vi "GetBit.vi"(8 "error in (no error)":errorcluster, 10 "Index":i32, 11 "Prime_Sieve in":refnum<class "Prime_Sieve.lvclass">) -> (0 "error out":errorcluster, 2 "Boolean":bool, 3 "Prime_Sieve out":refnum<class "Prime_Sieve.lvclass">)   [LabVIEW 2020, in "Prime_Sieve.lvclass"]
uses:
  Prime_Sieve.lvclass
  Prime_Sieve.lvclass/Prime_Sieve.ctl
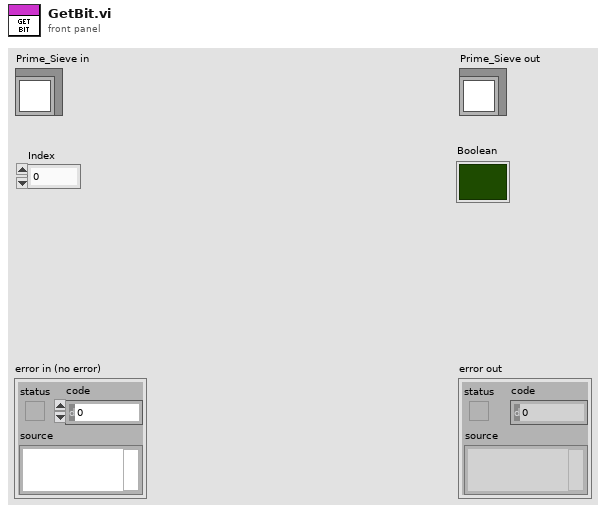
[diagram p1: front panel]
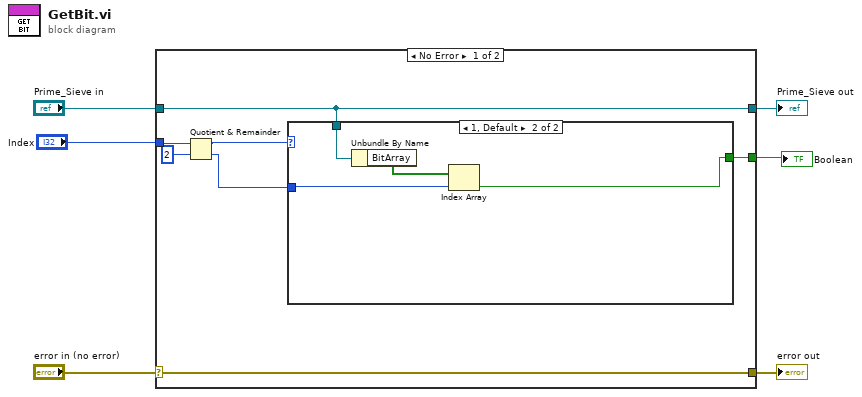
[diagram p0: block diagram]
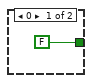
[diagram p2: hidden frame]
diagram:
  n1 = case shown="No Error" "error in (no error)" {
    selector: "error in (no error)" -> [w13 w20]
    tunnel: [w13 w20] -> w5
    tunnel: [w9 w19] -> w3
    tunnel: "Prime_Sieve in" -> [w9 w19]
    tunnel: "Index" -> [w12 _]
    tunnel: [w10 _] -> w1
    frame No Error {
      n2 = Quotient & Remainder(x=w12, y=2) -> (x-y*floor(x/y)=w8:i32, floor(x/y)=w7:i32)
      n3 = case shown="1, Default" w8 {
        tunnel: [FALSE w15] -> w10
        tunnel: w9 -> [_ w18]
        tunnel: w7 -> [_ w16]
        frame 0 {
        }
        frame 1, Default {
          n4 = Unbundle By Name(w18) -> ("BitArray"=w17:bool[])
          n5 = Index Array(array=w17, index=w16) -> (element=w15:bool)
        }
      }
    }
    frame Error {
    }
  }
  "error out" <- w5
  "Prime_Sieve out" <- w3
  "Boolean" <- w1
